vi "STAT2 decode ALL Analog data from Tool.vi"(0 "Received(T)":bool=TRUE, 5 "Selected Tool":T1, 7 "Controller SATT 2":T3 {"Tension Sub 2"."sys register" format="%04x"; "Tension Sub 1"."sys register" format="%04x"; "PSU"."sys register" format="%04x"; "solonoid"."valve status" format="%02x"; "solonoid"."sys register" format="%04x"; "pressure 2"."sys register" format="%04x"; "pressure 1"."sys register" format="%04x"; "Controller local"."High G monitoring" format="%02x"; "Controller local"."NA" format="%02x"; "Controller local"."GPIO values" format="%02x"; "Controller local"."Relay status" format="%02x"; "Controller local"."sys register" format="%04x"}, 11 "error in (no error)":errorcluster) -> (6 "Tool analog value":dbl[](array[numeric]), 8 "Analog for digital calc":T2, 10 "Tool analog index":u16[](array[numeric]), 15 "error out":errorcluster)   [LabVIEW 2011]
uses:
  Stroker/Stat def/Stroker system stat2.ctl
  LEINmaster/Nodes/Controller local stat2.ctl
  LEINmaster/Nodes/pressure stat2.ctl
  LEINmaster/Nodes/solonoid stat2.ctl
  LEINmaster/Nodes/PSU stat2.ctl
  LEINmaster/Nodes/tensionsub stat2.ctl
  Analog values for digital calculations.ctl
  List of tools.ctl
  Variable List Tool Analog.ctl
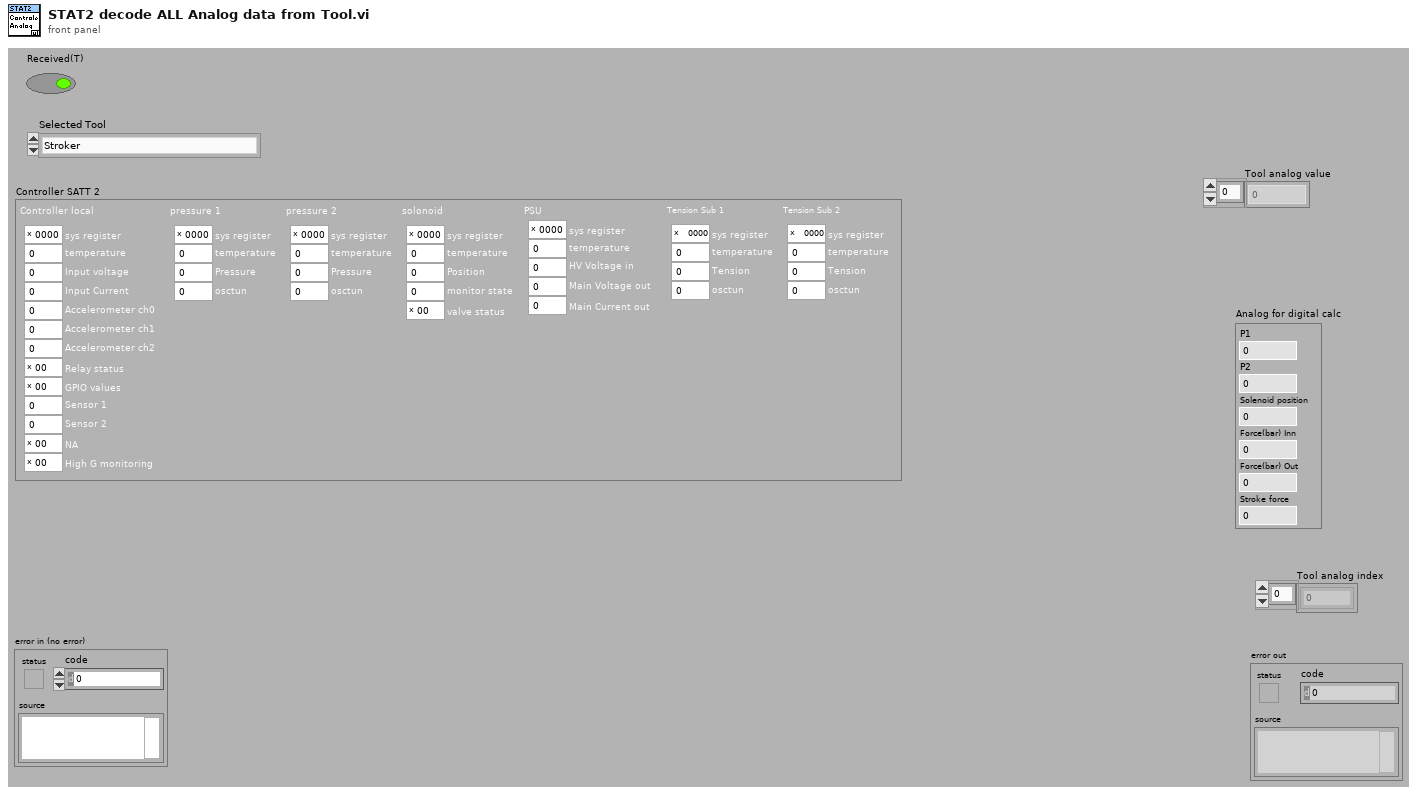
[diagram p1: front panel]
types:
  T1 = typedef "List of tools.ctl" = enum16{"Stroker", "Driller", "Tractor"}
  T2 = typedef "Analog values for digital calculations.ctl" = cluster{"P1":dbl, "P2":dbl, "Solenoid position":dbl, "Force(bar) Inn":dbl, "Force(bar) Out":dbl, "Stroke force":dbl}
  T3 = typedef "Stroker system stat2.ctl" = cluster{"Controller local":T4, "pressure 1":T5, "pressure 2":T5, "solonoid":T6, "PSU":T7, "Tension Sub 1":T8, "Tension Sub 2":T8}
  T4 = typedef "Controller local stat2.ctl" = cluster{"sys register":u16, "temperature":u16, "Input voltage":u16, "Input Current":u16, "Accelerometer ch0":u16, "Accelerometer ch1":u16, "Accelerometer ch2":u16, "Relay status":u8, "GPIO values":u8, "Sensor 1":i32, "Sensor 2":i32, "NA":u8, "High G monitoring":u8}
  T5 = typedef "pressure stat2.ctl" = cluster{"sys register":u16, "temperature":u16, "Pressure":u16, "osctun":u8}
  T6 = typedef "solonoid stat2.ctl" = cluster{"sys register":u16, "temperature":u16, "Position":i16, "monitor state":u8, "valve status":u8}
  T7 = typedef "PSU stat2.ctl" = cluster{"sys register":u16, "temperature":u16, "HV Voltage in":u16, "Main Voltage out":u16, "Main Current out":u16}
  T8 = typedef "tensionsub stat2.ctl" = cluster{"sys register":u16, "temperature":u16, "Tension":i16, "osctun":u8}
  T9 = typedef "Variable List Tool Analog.ctl" = enum16{"Tool Max Temperature", "Tool (Controller) Temperature", "Tool Supply Voltage", "Tool (Controller) Current", "Tool Acceleration X", "Tool Acceleration Y", "Tool Acceleration Z", "Tool Acceleration Sum", "Tool Inclination", "Tool Rotation", "Tool GP Sensor 1", "Tool GP Sensor 2", "Tool (Pressure 1) Temperature", "Tool Pressure 1 RAW", "Tool (Pressure 2) Temperature", "Tool Pressure 2 RAW", "Tool (Solenoid) Temperature", "Tool Solenoid Position", "PSU Temp", "Head Voltage", "PSU Main Voltage out", "PSU Main Current out", "Upper Tension Sub Temp", "Tool Upper Tension Sub Raw", "Lower Tension Sub Temp", "Tool Lower Tension Sub Raw", "Tool Var27 - Reserved", "Tool Var28 - Reserved", "Tool Var29 - Reserved", "Tool Var30 - Reserved", "Stroke Extension", "Stroke In Force", "Stroke Out Force", "Stroke Force", "Stroker Pressure 1", "Stroker Pressure 2", "Stroker Upper Tension Sub", "Stroker Lower Tension Sub", "Stroker Var09 - Reserved", "Stroker Var10 - Reserved", "Tractor Upper Tension Sub", "Tractor Lower Tension Sub", "Tractor Var03 - Reserved", "Tractor Var04 - Reserved", "Tool Temperature sensor", "Tool Motor Voltage", "Tool Motor Current", "Tool Motor Torque", "Tool weight on bit", "Tool Motor RPM"}
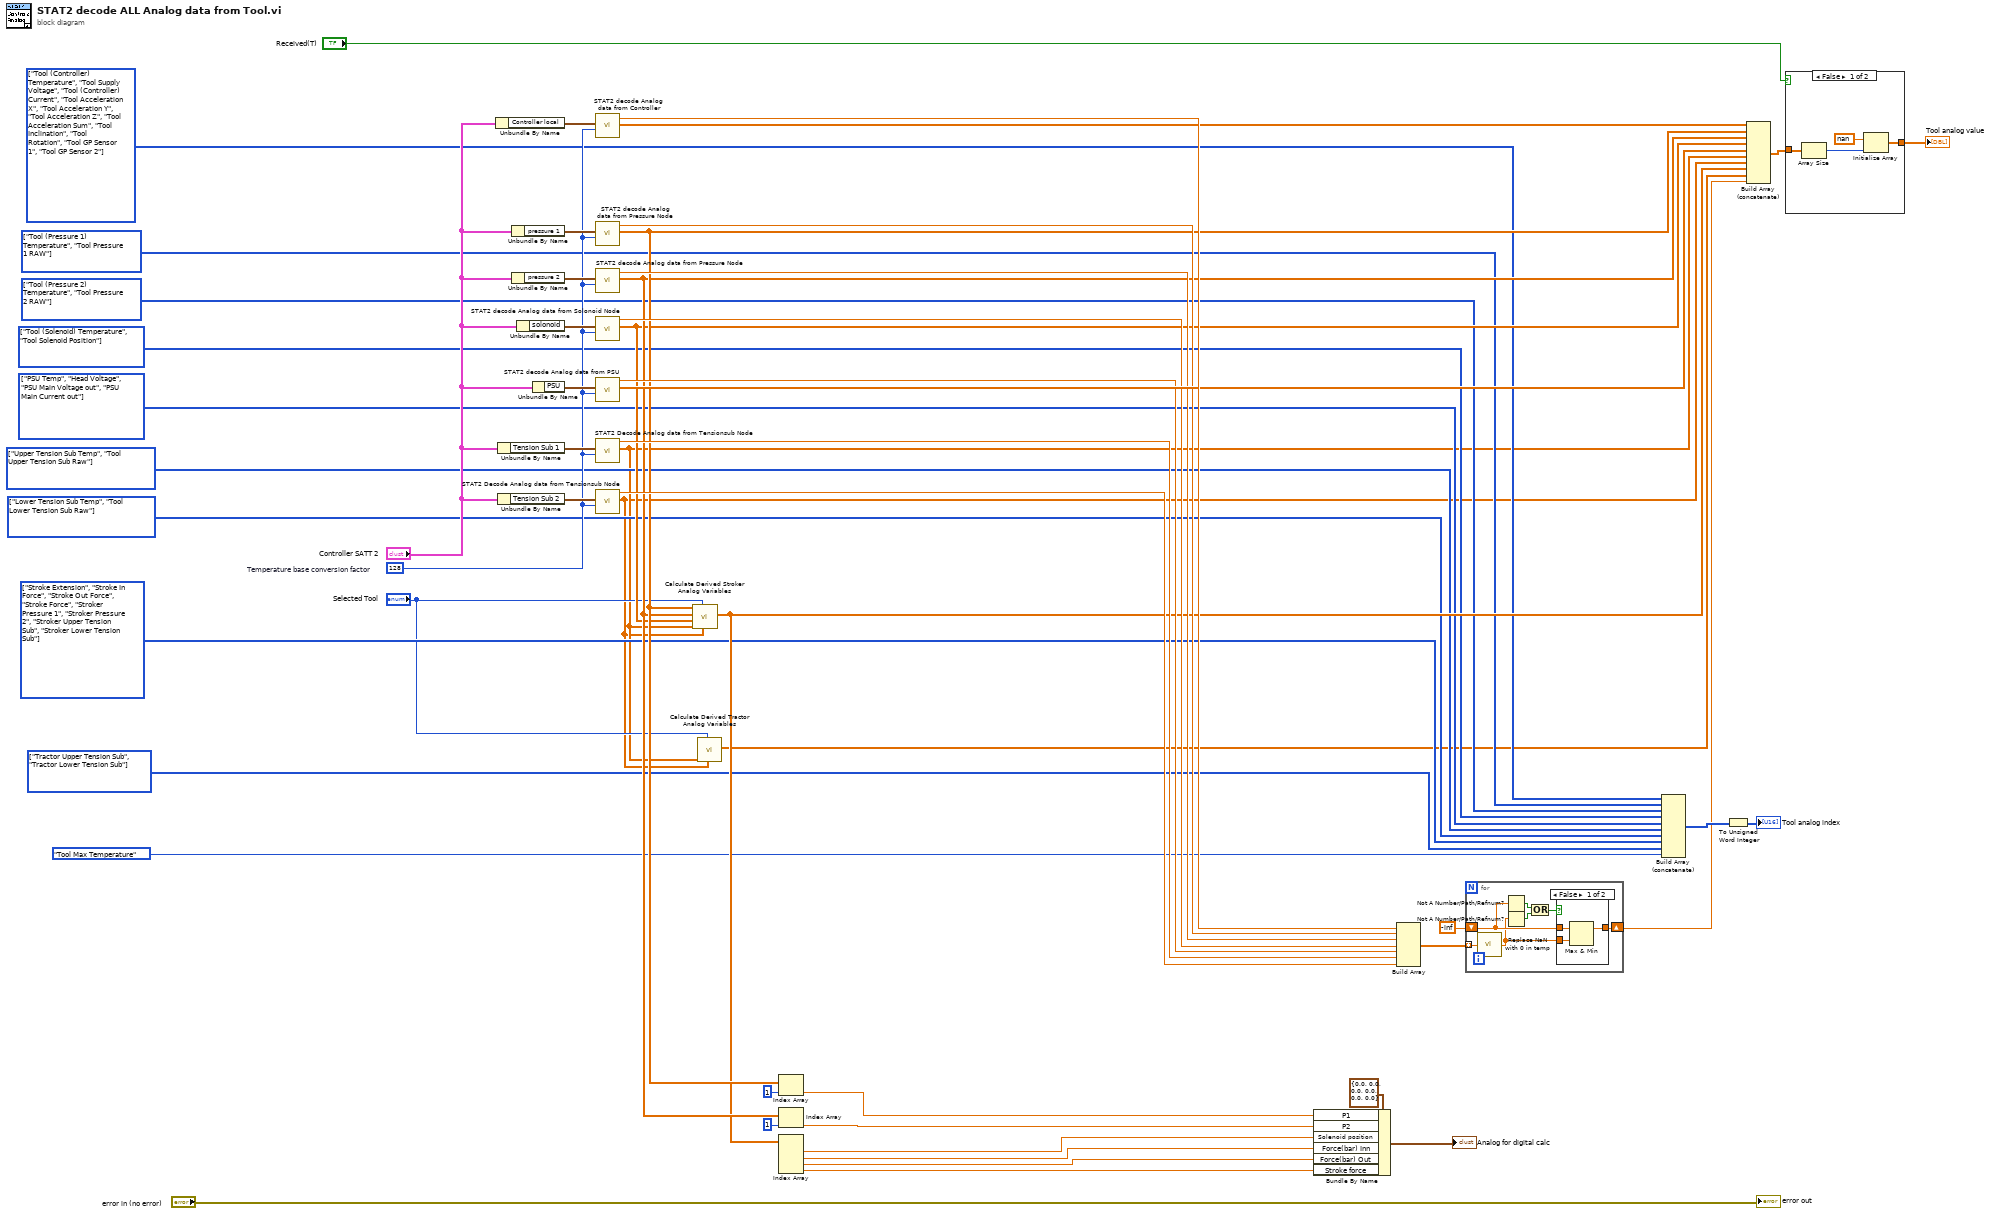
[diagram p0: block diagram]
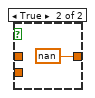
[diagram p2: hidden frame]
diagram:
  w3 = T9[] [enum."Tractor Upper Tension Sub", enum."Tractor Lower Tension Sub"] items=["Tool Max Temperature", "Tool (Controller) Temperature", "Tool Supply Voltage", "Tool (Controller) Current", "Tool Acceleration X", "Tool Acceleration Y", "Tool Acceleration Z", "Tool Acceleration Sum", "Tool Inclination", "Tool Rotation", "Tool GP Sensor 1", "Tool GP Sensor 2", "Tool (Pressure 1) Temperature", "Tool Pressure 1 RAW", "Tool (Pressure 2) Temperature", "Tool Pressure 2 RAW", "Tool (Solenoid) Temperature", "Tool Solenoid Position", "PSU Temp", "Head Voltage", "PSU Main Voltage out", "PSU Main Current out", "Upper Tension Sub Temp", "Tool Upper Tension Sub Raw", "Lower Tension Sub Temp", "Tool Lower Tension Sub Raw", "Tool Var27 - Reserved", "Tool Var28 - Reserved", "Tool Var29 - Reserved", "Tool Var30 - Reserved", "Stroke Extension", "Stroke In Force", "Stroke Out Force", "Stroke Force", "Stroker Pressure 1", "Stroker Pressure 2", "Stroker Upper Tension Sub", "Stroker Lower Tension Sub", "Stroker Var09 - Reserved", "Stroker Var10 - Reserved", "Tractor Upper Tension Sub", "Tractor Lower Tension Sub", "Tractor Var03 - Reserved", "Tractor Var04 - Reserved", "Tool Temperature sensor", "Tool Motor Voltage", "Tool Motor Current", "Tool Motor Torque", "Tool weight on bit", "Tool Motor RPM"]
  w15 = T9[] [enum."Stroke Extension", enum."Stroke In Force", enum."Stroke Out Force", enum."Stroke Force", enum."Stroker Pressure 1", enum."Stroker Pressure 2", enum."Stroker Upper Tension Sub", enum."Stroker Lower Tension Sub"] items=["Tool Max Temperature", "Tool (Controller) Temperature", "Tool Supply Voltage", "Tool (Controller) Current", "Tool Acceleration X", "Tool Acceleration Y", "Tool Acceleration Z", "Tool Acceleration Sum", "Tool Inclination", "Tool Rotation", "Tool GP Sensor 1", "Tool GP Sensor 2", "Tool (Pressure 1) Temperature", "Tool Pressure 1 RAW", "Tool (Pressure 2) Temperature", "Tool Pressure 2 RAW", "Tool (Solenoid) Temperature", "Tool Solenoid Position", "PSU Temp", "Head Voltage", "PSU Main Voltage out", "PSU Main Current out", "Upper Tension Sub Temp", "Tool Upper Tension Sub Raw", "Lower Tension Sub Temp", "Tool Lower Tension Sub Raw", "Tool Var27 - Reserved", "Tool Var28 - Reserved", "Tool Var29 - Reserved", "Tool Var30 - Reserved", "Stroke Extension", "Stroke In Force", "Stroke Out Force", "Stroke Force", "Stroker Pressure 1", "Stroker Pressure 2", "Stroker Upper Tension Sub", "Stroker Lower Tension Sub", "Stroker Var09 - Reserved", "Stroker Var10 - Reserved", "Tractor Upper Tension Sub", "Tractor Lower Tension Sub", "Tractor Var03 - Reserved", "Tractor Var04 - Reserved", "Tool Temperature sensor", "Tool Motor Voltage", "Tool Motor Current", "Tool Motor Torque", "Tool weight on bit", "Tool Motor RPM"]
  w8 = T9[] [enum."Lower Tension Sub Temp", enum."Tool Lower Tension Sub Raw"] items=["Tool Max Temperature", "Tool (Controller) Temperature", "Tool Supply Voltage", "Tool (Controller) Current", "Tool Acceleration X", "Tool Acceleration Y", "Tool Acceleration Z", "Tool Acceleration Sum", "Tool Inclination", "Tool Rotation", "Tool GP Sensor 1", "Tool GP Sensor 2", "Tool (Pressure 1) Temperature", "Tool Pressure 1 RAW", "Tool (Pressure 2) Temperature", "Tool Pressure 2 RAW", "Tool (Solenoid) Temperature", "Tool Solenoid Position", "PSU Temp", "Head Voltage", "PSU Main Voltage out", "PSU Main Current out", "Upper Tension Sub Temp", "Tool Upper Tension Sub Raw", "Lower Tension Sub Temp", "Tool Lower Tension Sub Raw", "Tool Var27 - Reserved", "Tool Var28 - Reserved", "Tool Var29 - Reserved", "Tool Var30 - Reserved", "Stroke Extension", "Stroke In Force", "Stroke Out Force", "Stroke Force", "Stroker Pressure 1", "Stroker Pressure 2", "Stroker Upper Tension Sub", "Stroker Lower Tension Sub", "Stroker Var09 - Reserved", "Stroker Var10 - Reserved", "Tractor Upper Tension Sub", "Tractor Lower Tension Sub", "Tractor Var03 - Reserved", "Tractor Var04 - Reserved", "Tool Temperature sensor", "Tool Motor Voltage", "Tool Motor Current", "Tool Motor Torque", "Tool weight on bit", "Tool Motor RPM"]
  w9 = T9[] [enum."Upper Tension Sub Temp", enum."Tool Upper Tension Sub Raw"] items=["Tool Max Temperature", "Tool (Controller) Temperature", "Tool Supply Voltage", "Tool (Controller) Current", "Tool Acceleration X", "Tool Acceleration Y", "Tool Acceleration Z", "Tool Acceleration Sum", "Tool Inclination", "Tool Rotation", "Tool GP Sensor 1", "Tool GP Sensor 2", "Tool (Pressure 1) Temperature", "Tool Pressure 1 RAW", "Tool (Pressure 2) Temperature", "Tool Pressure 2 RAW", "Tool (Solenoid) Temperature", "Tool Solenoid Position", "PSU Temp", "Head Voltage", "PSU Main Voltage out", "PSU Main Current out", "Upper Tension Sub Temp", "Tool Upper Tension Sub Raw", "Lower Tension Sub Temp", "Tool Lower Tension Sub Raw", "Tool Var27 - Reserved", "Tool Var28 - Reserved", "Tool Var29 - Reserved", "Tool Var30 - Reserved", "Stroke Extension", "Stroke In Force", "Stroke Out Force", "Stroke Force", "Stroker Pressure 1", "Stroker Pressure 2", "Stroker Upper Tension Sub", "Stroker Lower Tension Sub", "Stroker Var09 - Reserved", "Stroker Var10 - Reserved", "Tractor Upper Tension Sub", "Tractor Lower Tension Sub", "Tractor Var03 - Reserved", "Tractor Var04 - Reserved", "Tool Temperature sensor", "Tool Motor Voltage", "Tool Motor Current", "Tool Motor Torque", "Tool weight on bit", "Tool Motor RPM"]
  w10 = T9[] [enum."PSU Temp", enum."Head Voltage", enum."PSU Main Voltage out", enum."PSU Main Current out"] items=["Tool Max Temperature", "Tool (Controller) Temperature", "Tool Supply Voltage", "Tool (Controller) Current", "Tool Acceleration X", "Tool Acceleration Y", "Tool Acceleration Z", "Tool Acceleration Sum", "Tool Inclination", "Tool Rotation", "Tool GP Sensor 1", "Tool GP Sensor 2", "Tool (Pressure 1) Temperature", "Tool Pressure 1 RAW", "Tool (Pressure 2) Temperature", "Tool Pressure 2 RAW", "Tool (Solenoid) Temperature", "Tool Solenoid Position", "PSU Temp", "Head Voltage", "PSU Main Voltage out", "PSU Main Current out", "Upper Tension Sub Temp", "Tool Upper Tension Sub Raw", "Lower Tension Sub Temp", "Tool Lower Tension Sub Raw", "Tool Var27 - Reserved", "Tool Var28 - Reserved", "Tool Var29 - Reserved", "Tool Var30 - Reserved", "Stroke Extension", "Stroke In Force", "Stroke Out Force", "Stroke Force", "Stroker Pressure 1", "Stroker Pressure 2", "Stroker Upper Tension Sub", "Stroker Lower Tension Sub", "Stroker Var09 - Reserved", "Stroker Var10 - Reserved", "Tractor Upper Tension Sub", "Tractor Lower Tension Sub", "Tractor Var03 - Reserved", "Tractor Var04 - Reserved", "Tool Temperature sensor", "Tool Motor Voltage", "Tool Motor Current", "Tool Motor Torque", "Tool weight on bit", "Tool Motor RPM"]
  w11 = T9[] [enum."Tool (Solenoid) Temperature", enum."Tool Solenoid Position"] items=["Tool Max Temperature", "Tool (Controller) Temperature", "Tool Supply Voltage", "Tool (Controller) Current", "Tool Acceleration X", "Tool Acceleration Y", "Tool Acceleration Z", "Tool Acceleration Sum", "Tool Inclination", "Tool Rotation", "Tool GP Sensor 1", "Tool GP Sensor 2", "Tool (Pressure 1) Temperature", "Tool Pressure 1 RAW", "Tool (Pressure 2) Temperature", "Tool Pressure 2 RAW", "Tool (Solenoid) Temperature", "Tool Solenoid Position", "PSU Temp", "Head Voltage", "PSU Main Voltage out", "PSU Main Current out", "Upper Tension Sub Temp", "Tool Upper Tension Sub Raw", "Lower Tension Sub Temp", "Tool Lower Tension Sub Raw", "Tool Var27 - Reserved", "Tool Var28 - Reserved", "Tool Var29 - Reserved", "Tool Var30 - Reserved", "Stroke Extension", "Stroke In Force", "Stroke Out Force", "Stroke Force", "Stroker Pressure 1", "Stroker Pressure 2", "Stroker Upper Tension Sub", "Stroker Lower Tension Sub", "Stroker Var09 - Reserved", "Stroker Var10 - Reserved", "Tractor Upper Tension Sub", "Tractor Lower Tension Sub", "Tractor Var03 - Reserved", "Tractor Var04 - Reserved", "Tool Temperature sensor", "Tool Motor Voltage", "Tool Motor Current", "Tool Motor Torque", "Tool weight on bit", "Tool Motor RPM"]
  w12 = T9[] [enum."Tool (Pressure 2) Temperature", enum."Tool Pressure 2 RAW"] items=["Tool Max Temperature", "Tool (Controller) Temperature", "Tool Supply Voltage", "Tool (Controller) Current", "Tool Acceleration X", "Tool Acceleration Y", "Tool Acceleration Z", "Tool Acceleration Sum", "Tool Inclination", "Tool Rotation", "Tool GP Sensor 1", "Tool GP Sensor 2", "Tool (Pressure 1) Temperature", "Tool Pressure 1 RAW", "Tool (Pressure 2) Temperature", "Tool Pressure 2 RAW", "Tool (Solenoid) Temperature", "Tool Solenoid Position", "PSU Temp", "Head Voltage", "PSU Main Voltage out", "PSU Main Current out", "Upper Tension Sub Temp", "Tool Upper Tension Sub Raw", "Lower Tension Sub Temp", "Tool Lower Tension Sub Raw", "Tool Var27 - Reserved", "Tool Var28 - Reserved", "Tool Var29 - Reserved", "Tool Var30 - Reserved", "Stroke Extension", "Stroke In Force", "Stroke Out Force", "Stroke Force", "Stroker Pressure 1", "Stroker Pressure 2", "Stroker Upper Tension Sub", "Stroker Lower Tension Sub", "Stroker Var09 - Reserved", "Stroker Var10 - Reserved", "Tractor Upper Tension Sub", "Tractor Lower Tension Sub", "Tractor Var03 - Reserved", "Tractor Var04 - Reserved", "Tool Temperature sensor", "Tool Motor Voltage", "Tool Motor Current", "Tool Motor Torque", "Tool weight on bit", "Tool Motor RPM"]
  w13 = T9[] [enum."Tool (Pressure 1) Temperature", enum."Tool Pressure 1 RAW"] items=["Tool Max Temperature", "Tool (Controller) Temperature", "Tool Supply Voltage", "Tool (Controller) Current", "Tool Acceleration X", "Tool Acceleration Y", "Tool Acceleration Z", "Tool Acceleration Sum", "Tool Inclination", "Tool Rotation", "Tool GP Sensor 1", "Tool GP Sensor 2", "Tool (Pressure 1) Temperature", "Tool Pressure 1 RAW", "Tool (Pressure 2) Temperature", "Tool Pressure 2 RAW", "Tool (Solenoid) Temperature", "Tool Solenoid Position", "PSU Temp", "Head Voltage", "PSU Main Voltage out", "PSU Main Current out", "Upper Tension Sub Temp", "Tool Upper Tension Sub Raw", "Lower Tension Sub Temp", "Tool Lower Tension Sub Raw", "Tool Var27 - Reserved", "Tool Var28 - Reserved", "Tool Var29 - Reserved", "Tool Var30 - Reserved", "Stroke Extension", "Stroke In Force", "Stroke Out Force", "Stroke Force", "Stroker Pressure 1", "Stroker Pressure 2", "Stroker Upper Tension Sub", "Stroker Lower Tension Sub", "Stroker Var09 - Reserved", "Stroker Var10 - Reserved", "Tractor Upper Tension Sub", "Tractor Lower Tension Sub", "Tractor Var03 - Reserved", "Tractor Var04 - Reserved", "Tool Temperature sensor", "Tool Motor Voltage", "Tool Motor Current", "Tool Motor Torque", "Tool weight on bit", "Tool Motor RPM"]
  w14 = T9[] [enum."Tool (Controller) Temperature", enum."Tool Supply Voltage", enum."Tool (Controller) Current", enum."Tool Acceleration X", enum."Tool Acceleration Y", enum."Tool Acceleration Z", enum."Tool Acceleration Sum", enum."Tool Inclination", enum."Tool Rotation", enum."Tool GP Sensor 1", enum."Tool GP Sensor 2"] items=["Tool Max Temperature", "Tool (Controller) Temperature", "Tool Supply Voltage", "Tool (Controller) Current", "Tool Acceleration X", "Tool Acceleration Y", "Tool Acceleration Z", "Tool Acceleration Sum", "Tool Inclination", "Tool Rotation", "Tool GP Sensor 1", "Tool GP Sensor 2", "Tool (Pressure 1) Temperature", "Tool Pressure 1 RAW", "Tool (Pressure 2) Temperature", "Tool Pressure 2 RAW", "Tool (Solenoid) Temperature", "Tool Solenoid Position", "PSU Temp", "Head Voltage", "PSU Main Voltage out", "PSU Main Current out", "Upper Tension Sub Temp", "Tool Upper Tension Sub Raw", "Lower Tension Sub Temp", "Tool Lower Tension Sub Raw", "Tool Var27 - Reserved", "Tool Var28 - Reserved", "Tool Var29 - Reserved", "Tool Var30 - Reserved", "Stroke Extension", "Stroke In Force", "Stroke Out Force", "Stroke Force", "Stroker Pressure 1", "Stroker Pressure 2", "Stroker Upper Tension Sub", "Stroker Lower Tension Sub", "Stroker Var09 - Reserved", "Stroker Var10 - Reserved", "Tractor Upper Tension Sub", "Tractor Lower Tension Sub", "Tractor Var03 - Reserved", "Tractor Var04 - Reserved", "Tool Temperature sensor", "Tool Motor Voltage", "Tool Motor Current", "Tool Motor Torque", "Tool weight on bit", "Tool Motor RPM"]
  w36 = u16 128  # Temperature base conversion factor
  n1 = Unbundle By Name("Controller SATT 2") -> ("Controller local"=w45:T4)
  n2 = Unbundle By Name("Controller SATT 2") -> ("Tension Sub 1"=w43:T8)
  n3 = Unbundle By Name("Controller SATT 2") -> ("Tension Sub 2"=w38:T8)
  n4 = Unbundle By Name("Controller SATT 2") -> ("pressure 1"=w42:T5)
  n5 = Unbundle By Name("Controller SATT 2") -> ("pressure 2"=w41:T5)
  n6 = Unbundle By Name("Controller SATT 2") -> ("solonoid"=w37:T6)
  n7 = Unbundle By Name("Controller SATT 2") -> ("PSU"=w44:T7)
  n8 = call "STAT2 decode Analog data from Controller.vi"("Temperature base conversion factor"=w36, "Controller local"=w45) -> ("Controller analog data"=w35:dbl[], "Temperature"=w46:dbl)  [unwired: 8 in]
  n9 = call "STAT2 decode Analog data from Pressure Node.vi"("Temperature base conversion factor"=w36, "Pressure"=w42) -> ("Node Analog value"=w26:dbl[], "Temperature"=w32:dbl)  [unwired: 8 in]
  n10 = call "STAT2 decode Analog data from Pressure Node.vi"("Temperature base conversion factor"=w36, "Pressure"=w41) -> ("Node Analog value"=w25:dbl[], "Temperature"=w31:dbl)  [unwired: 8 in]
  n11 = call "STAT2 decode Analog data from Solonoid Node.vi"("Temperature base conversion factor"=w36, "Solonoid"=w37) -> ("Node Analog value"=w24:dbl[], "Temperature"=w30:dbl)  [unwired: 8 in]
  n12 = call "STAT2 decode Analog data from PSU.vi"("Temperature base conversion factor"=w36, "PSU"=w44) -> ("Node Analog value"=w34:dbl[], "Temperature"=w29:dbl)  [unwired: 8 in]
  n13 = call "STAT2 Decode Analog data from Tensionsub Node.vi"("Temperature base conversion factor"=w36, "Tension Sub"=w43) -> ("Node Analog value"=w6:dbl[], "Temperature"=w28:dbl)  [unwired: 8 in]
  n14 = call "STAT2 Decode Analog data from Tensionsub Node.vi"("Temperature base conversion factor"=w36, "Tension Sub"=w38) -> ("Node Analog value"=w5:dbl[], "Temperature"=w27:dbl)  [unwired: 8 in]
  n15 = call "Calculate Derived Stroker Analog Variables.vi"("Lower Tension Sub Data"=w5, "Selected Tool"="Selected Tool", "Upper Tension Sub Data"=w6, "Solenoid Analog Data"=w24, "Pressure 2 Analog Data"=w25, "Pressure 1 Analog Data"=w26) -> ("Stroker Data Out"=w16:dbl[])  [unwired: 5 in]
  n16 = call "Calculate Derived Tractor Analog Variables.vi"("Lower Tension Sub Data"=w5, "Selected Tool"="Selected Tool", "Upper Tension Sub Data"=w6) -> ("Stroker Data Out"=w2:dbl[])  [unwired: 8 in]
  n17 = Index Array(array=w26, index=1) -> (element=w22:dbl)
  n18 = Index Array(array=w25, index=1) -> (element=w21:dbl)
  n19 = Index Array(array=w16) -> (element #1=w20:dbl, element #2=w19:dbl, element #3=w18:dbl, element #4=w17:dbl)  [unwired: 4 in]
  n20 = Bundle By Name(cluster=T2 {"P1"=0.0, "P2"=0.0, "Solenoid position"=0.0, "Force(bar) Inn"=0.0, "Force(bar) Out"=0.0, "Stroke force"=0.0} ("Analog for digital calc"), "P1"=w22, "P2"=w21, "Solenoid position"=w20, "Force(bar) Inn"=w19, "Force(bar) Out"=w18, "Stroke force"=w17) -> (→"Analog for digital calc":T2)
  n21 = Build Array(w46, w32, w31, w30, w29, w28, w27) -> (w51:dbl[])
  n22 = for {
    tunnel: w51 -> [w57] mode=indexing
    shift-right: [w62] -> w1
    shift-left: -inf -> [w61]
    n23 = call "Replace NaN with 0 in temp.vi"("Temperature in"=w57) -> ("Temperature out"=w56:dbl)  [unwired: 14 in]
    n24 = Not A Number/Path/Refnum?(number/path/refnum=w61) -> (NaN/Path/Refnum?=w59:bool)
    n25 = Not A Number/Path/Refnum?(number/path/refnum=w56) -> (NaN/Path/Refnum?=w60:bool)
    n26 = Or(x=w59, y=w60) -> (x .or. y?=w58:bool)
    n27 = case shown="False" w58 {
      tunnel: [w65 nan] -> w62
      tunnel: w61 -> [w64 _]
      tunnel: w56 -> [w63 _]
      frame False {
        n28 = Max & Min(x=w64, y=w63) -> (max(x,y)=w65:dbl)  [unwired: 1 out]
      }
      frame True {
      }
    }
  }
  n29 = Build Array (concatenate)(w14, w13, w12, w11, w10, w9, w8, w15, w3, Variable_List_Tool_Analog."Tool Max Temperature" ("Variable ID")) -> (w55:T9[])
  n30 = To Unsigned Word Integer(number=w55) -> (unsigned 16bit integer=→"Tool analog index":u16[])
  n31 = Build Array (concatenate)(w35, w26, w25, w24, w34, w6, w5, w16, w2, w1) -> (w52:dbl[])
  n32 = case shown="False" "Received(T)" {
    tunnel: [w67 w71] -> w53
    tunnel: w52 -> [w70 w71]
    frame False {
      n33 = Array Size(array=w70) -> (size(s)=w69:i32)
      n34 = Initialize Array(nan ("element"), w69) -> (w67:dbl[])
    }
    frame True {
    }
  }
  "Tool analog value" <- w53
  "error out" <- "error in (no error)"
